vi "Index Array (Boolean).vi"(8 "error in (no error)":errorcluster, 9 "index":i32, 10 "JSON Value in":refnum<class "JSON Value.lvclass">) -> (0 "error out":errorcluster, 1 "Boolean":bool)   [LabVIEW 2016, in "JSON Value.lvclass"]
doc: "Returns the Boolean value of the JSON Boolean element of the JSON array at index."
uses:
  JSON Value.lvclass
  Read Value/Read value (Boolean).vi
  Index Array (Value).vi
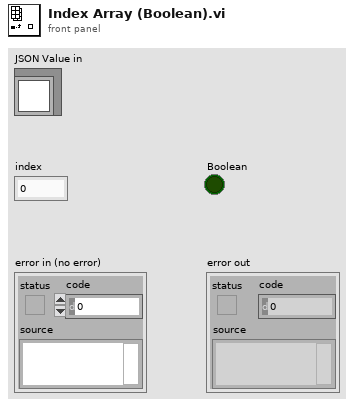
[diagram p1: front panel]
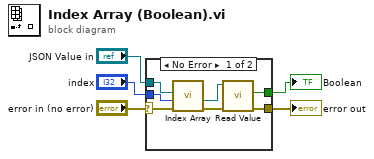
[diagram p0: block diagram]
diagram:
  n1 = case shown="No Error" "error in (no error)" {
    selector: "error in (no error)" -> [w8 w13]
    tunnel: [w9 w13] -> w5
    tunnel: "JSON Value in" -> [w7 _]
    tunnel: "index" -> [w6 _]
    tunnel: [w10 _] -> w3
    frame No Error {
      n2 = call-poly "Index Array.vi"("error in"=w8, "index"=w6, "JSON Value in"=w7) -> ("error out"=w11:errorcluster, "JSON Value out"=w12:refnum<class "JSON Value.lvclass">)  [unwired: 7 in]
      n3 = call-poly "Read Value.vi"("error in (no error)"=w11, "JSON Boolean in"=w12) -> ("error out"=w9:errorcluster, "value"=w10:bool)  [unwired: 7 in, 1 out]
    }
    frame Error {
    }
  }
  "error out" <- w5
  "Boolean" <- w3
